vi "Panel Scale Reading Percision.vi"(0 "VISA resource name":refnum<visa-resource-name>="COM1") -> (4 "read buffer":string)   [LabVIEW 2012]
uses:
  <vilib>/Instr/_visa.llb/VISA Configure Serial Port (Instr).vi
panel:
  in  "overide":bool
  out "Stable":bool
  out "error out":errorcluster
  in  "Zero":bool=TRUE
  in  "stop":bool
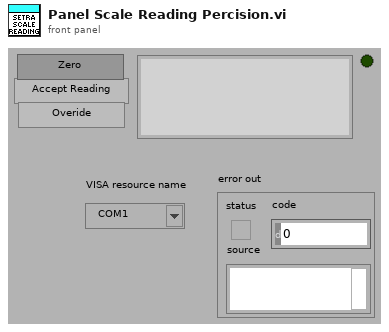
[diagram p1: front panel]
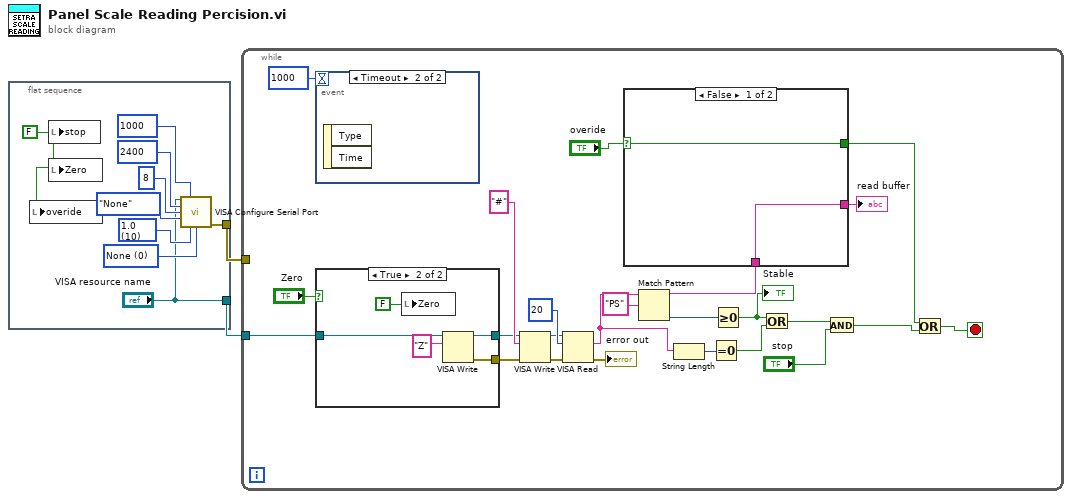
[diagram p0: block diagram]
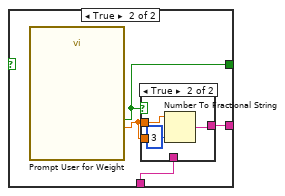
[diagram p2: hidden frame]
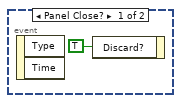
[diagram p4: hidden frame]
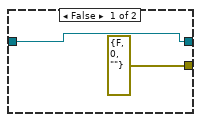
[diagram p5: hidden frame]
diagram:
  n1 = flat-sequence {
    tunnel: [w5] -> w2
    tunnel: ["VISA resource name"] -> w1
    frame #0 {
      w3 = FALSE ("Zero")
      w7 = u16 0 items=["None", "XON/XOFF", "RTS/CTS", "XON/XOFF & RTS/CTS", "DTR/DSR", "XON/XOFF & DTR/DSR"] ("flow control (0:none)")
      w8 = u16 10 items=["1.0"=10, "1.5"=15, "2.0"=20] ("stop bits (10: 1 bit)")
      n2 = local write "overide"(w3) -> ()
      n3 = local write "stop"(w3) -> ()
      n4 = local write "Zero"(w3) -> ()
      n5 = call-poly "VISA Configure Serial Port"("VISA resource name"="VISA resource name", "timeout (10sec)"=u32 1000, "baud rate (9600)"=u32 2400, "data bits (8)"=u16 8, "parity (0:none)"=enum16{"None", "Odd", "Even", "Mark", "Space"}."None", "stop bits (10: 1 bit)"=w8, "flow control (0:none)"=w7) -> ("error out"=w5:errorcluster)  [unwired: 7 in, 1 out]
    }
  }
  n6 = while {
    tunnel: w2 -> [_]
    tunnel: w1 -> [w34]
    stop <- w15 stop-if-true
    n7 = event shown="[1] Timeout" {
      selector: _ -> [_ _]
      dyn-events: _ -> [_ _]
      timeout: 1000 ("millisecond multiple") -> [_ _]
      event Panel Close? {
        n8 = event-data() -> ()  [unwired: 1 in, 2 out]
        n9 = event-data("Discard?"=TRUE) -> ()  [unwired: 1 in, 1 out]
      }
      event Timeout {
        n10 = event-data() -> ()  [unwired: 1 in, 2 out]
      }
    }
    n11 = case shown="True" "Zero" {
      tunnel: w34 -> [w48 w53]
      tunnel: [w48 w51] -> w29
      tunnel: [errorcluster {"status"=FALSE, "code"=0, "source"=""} ("error out") w50] -> w28
      frame False {
      }
      frame True {
        n12 = local write "Zero"(FALSE ("Zero")) -> ()
        n13 = VISA Write(VISA resource name=w53, write buffer="Z") -> (VISA resource name out=w51:refnum<visa-resource-name>, error out=w50:errorcluster)  [unwired: 1 in, 1 out]
      }
    }
    n14 = VISA Write(VISA resource name=w29, write buffer="#", error in (no error)=w28) -> (VISA resource name out=w31:refnum<visa-resource-name>, error out=w30:errorcluster)  [unwired: 1 out]
    n15 = VISA Read(VISA resource name=w31, byte count=u32 20, error in (no error)=w30) -> (read buffer=w18:string, error out=→"error out":errorcluster)  [unwired: 2 out]
    n16 = Match Pattern(string=w18, regular expression="PS") -> (before substring=w12:string, offset past match=w25:i32)  [unwired: 1 in, 2 out]
    n17 = case shown="False" "overide" {
      selector: "overide" -> [w37 _]
      tunnel: [w37 w40] -> w14
      tunnel: [w36 w41] -> w13
      tunnel: w12 -> [w36 w39]
      frame False {
      }
      frame True {
        n18 = call "Prompt User for Weight"() -> ("Weight"=w38:dbl, "OK"=w40:bool)  [unwired: 17 in, 1 out]
        n19 = case shown="True" w40 {
          tunnel: [w42 w45] -> w41
          tunnel: w38 -> [_ w44]
          tunnel: w39 -> [w42 _]
          tunnel: w38 -> [_ _]
          frame False {
          }
          frame True {
            n20 = Number To Fractional String(number=w44, precision (6)=i16 3) -> (F-format string=w45:string)  [unwired: 2 in]
          }
        }
      }
    }
    "read buffer" <- w13
    n21 = String Length(string=w18) -> (length=w19:i32)
    n22 = Equal To 0?(x=w19) -> (x = 0?=w17:bool)
    n23 = Greater Or Equal To 0?(x=w25) -> (x >= 0?=w22:bool)
    "Stable" <- w22
    n24 = Or(x=w22, y=w17) -> (x .or. y?=w20:bool)
    n25 = And(x=w20, y="stop") -> (x .and. y?=w23:bool)
    n26 = Or(x=w14, y=w23) -> (x .or. y?=w15:bool)
  }
